vi "_FPGA Send LCD.vi"(5 "error in (no error)":errorcluster, 6 "Message":string, 7 "Command":T1) -> (0 "error out":errorcluster, 1 "Key Pressed":bool, 2 "Reply":string)   [LabVIEW 2012]
uses:
  Type/_RT LED Num.ctl
  Type/_RT Serial Command.ctl
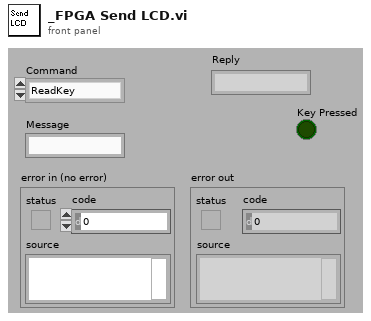
[diagram p1: front panel]
types:
  T1 = typedef "_RT LED Num.ctl" = enum8{"ReadKey", "ClearKeyBuffer", "ClearLCD", "BacklightOn"}
  T2 = typedef "_RT Serial Command.ctl" = cluster{"Port Type":u16, "baud rate (9600)":u32, "data bits (8)":u16, "stop bits (1)":u16, "parity (0:none)":u16, "DoRead":bool, "Command":string}
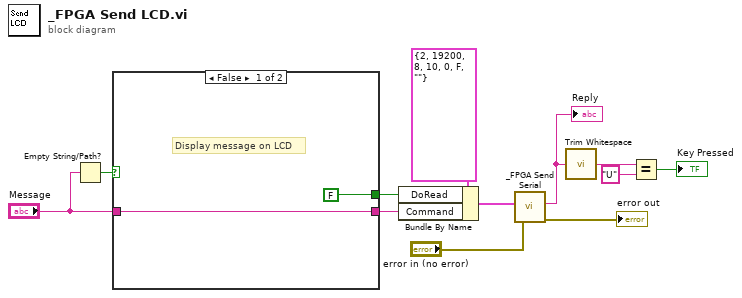
[diagram p0: block diagram]
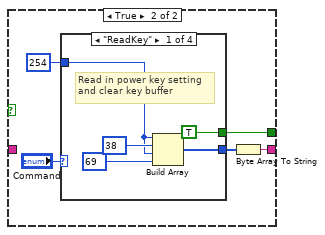
[diagram p2: hidden frame]
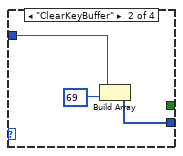
[diagram p3: hidden frame]
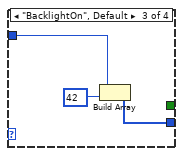
[diagram p4: hidden frame]
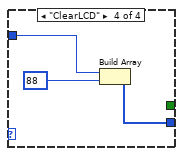
[diagram p5: hidden frame]
diagram:
  n1 = Empty String/Path?(string/path="Message") -> (empty?=w10:bool)
  n2 = case shown="False" w10 {
    tunnel: [w14 w19] -> w8
    tunnel: "Message" -> [w14 _]
    tunnel: [FALSE w15] -> w6
    frame False {
      # "Display message on LCD"
    }
    frame True {
      n3 = case shown="\"ReadKey\"" "Command" {
        tunnel: u8 254 -> [w22 w27 w30 w32]
        tunnel: [w20 w25 w28 w33] -> w16
        tunnel: [TRUE _ _ _] -> w15
        frame "ReadKey" {
          # "Read in power key setting\nand clear key buffer"
          n4 = Build Array(w22, u8 38, w22, u8 69) -> (w20:u8[])
        }
        frame "ClearKeyBuffer" {
          n5 = Build Array(w27, u8 69) -> (w25:u8[])
        }
        frame "BacklightOn", Default {
          n6 = Build Array(w30, u8 42) -> (w28:u8[])
        }
        frame "ClearLCD" {
          n7 = Build Array(w32, u8 88) -> (w33:u8[])
        }
      }
      n8 = Byte Array To String(unsigned byte array=w16) -> (string=w19:string)
    }
  }
  n9 = Bundle By Name(cluster=T2 {"Port Type"=2, "baud rate (9600)"=19200, "data bits (8)"=8, "stop bits (1)"=10, "parity (0:none)"=0, "DoRead"=FALSE, "Command"=""} ("Serial Command"), "DoRead"=w6, "Command"=w8) -> (w12:T2)
  n10 = call "_FPGA Send Serial.vi"("error in"="error in (no error)", "Serial Command"=w12) -> ("error out"=→"error out":errorcluster, "Reply"=w7:string)  [unwired: 2 in, 2 out]
  "Reply" <- w7
  n11 = call <vilib>:"Trim Whitespace.vi"("string"=w7) -> ("trimmed string"=w2:string)  [unwired: 1 in]
  n12 = Equal?(x=w2, y="U") -> (x = y?=→"Key Pressed":bool)
